vi "Simple Playback Controller.vi"() -> ()   [LabVIEW 2010]
panel:
  out "Joint States":T1(array[cluster])
  in  "Play":bool
  out "Array":T2(array[cluster])
  in  "Done":bool
  in  "Script of positions":i32(listbox)
  in  "Add":bool
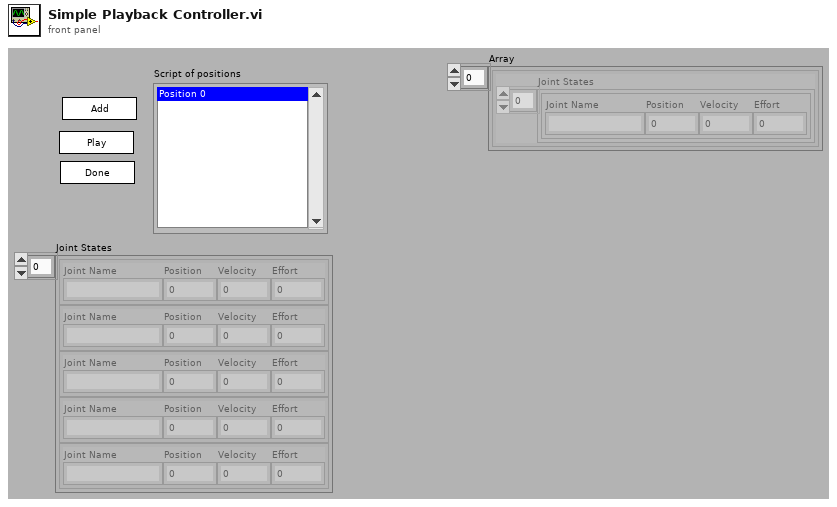
[diagram p1: front panel]
types:
  T1 = cluster{"Joint Name":string, "Position":dbl, "Velocity":dbl, "Effort":dbl}[]
  T2 = cluster{"Joint States":cluster{"Joint Name":string, "Position":dbl, "Velocity":dbl, "Effort":dbl}[]}[]
  T3 = cluster{"Joint States":cluster{"Joint Name":string, "Position":dbl, "Velocity":dbl, "Effort":dbl}[]}
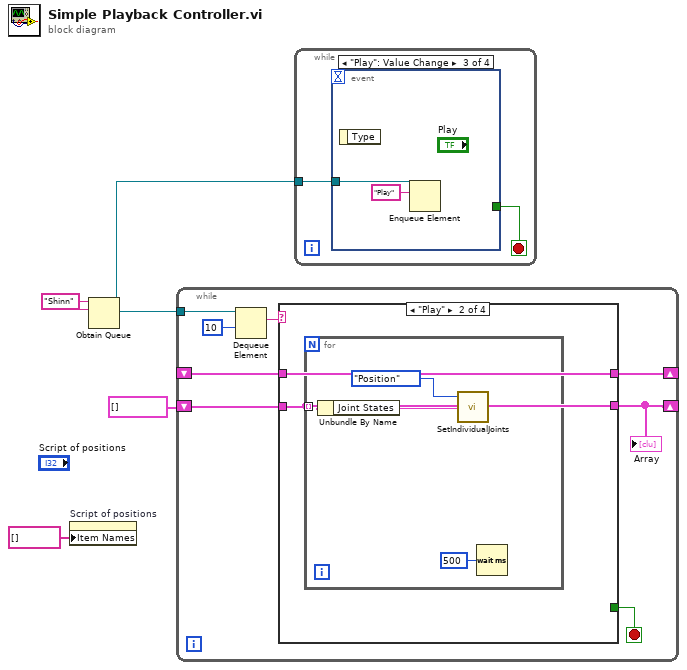
[diagram p0: block diagram]
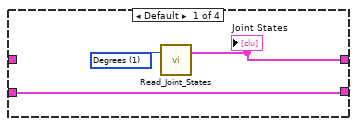
[diagram p2: hidden frame]
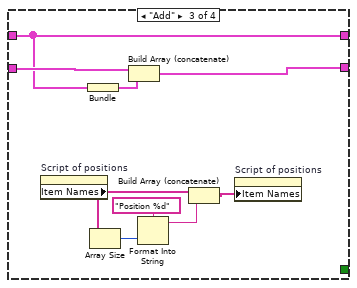
[diagram p3: hidden frame]
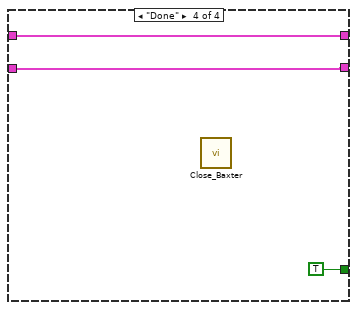
[diagram p4: hidden frame]
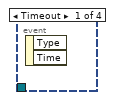
[diagram p5: hidden frame]
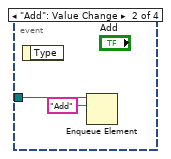
[diagram p6: hidden frame]
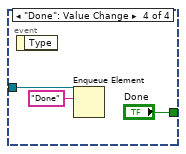
[diagram p7: hidden frame]
diagram:
  w4 = "Shinn" ("name (unnamed)")
  n1 = property on="Script of positions" class="LstBox (strict)"("Item Names"=string[] []) -> ()  [unwired: 2 in, 2 out]
  n2 = Obtain Queue(name (unnamed)=w4, element data type=w4) -> (queue out=w3:refnum<queue>)  [unwired: 3 in, 2 out]
  n3 = while {
    tunnel: w3 -> [w12]
    shift-right: [w8] -> _
    shift-left: _ -> [w7]
    shift-right: [w5] -> _
    shift-left: T2 [] -> [w6]
    stop <- w10 stop-if-true
    n4 = Dequeue Element(queue=w12, timeout in ms (-1)=10) -> (element=w11:string)  [unwired: 1 in, 3 out]
    n5 = case shown="\"Play\"" w11 {
      tunnel: [_ _ _ TRUE] -> w10
      tunnel: [w14 w17 w22 w32] -> w8
      tunnel: w7 -> [_ w17 w22 w32]
      tunnel: [w13 w16 w30 w31] -> w5
      tunnel: w6 -> [w13 w16 w29 w31]
      frame Default {
        w15 = u16 1 items=["Radians", "Degrees"] ("Units (Rad)")
        n6 = call <userlib>:"Read_Joint_States.vi"("Units (deg)"=w15) -> ("Joint States"=w14:T1)  [unwired: 2 in, 1 out]
        "Joint States" <- w14
      }
      frame "Play" {
        n7 = for {
          tunnel: w16 -> [w19] mode=indexing
          n8 = Unbundle By Name(w19) -> ("Joint States"=w18:T1)
          n9 = call <userlib>:"SetIndividualJoints.vi"("Mode"=enum16{"Position", "Velocity", "Effort"}."Position", "Joint States"=w18) -> ()  [unwired: 4 in, 1 out]
          n10 = Wait (ms)(milliseconds to wait=u32 500) -> ()  [unwired: 1 out]
        }
      }
      frame "Add" {
        n11 = property on="Script of positions" class="LstBox (strict)"() -> ("Item Names"=w25:string[])  [unwired: 2 in, 2 out]
        n12 = Bundle("Joint States"=w22) -> (w23:T3)  [unwired: 1 in]
        n13 = Array Size(array=w25) -> (size(s)=w26:i32)
        n14 = Build Array (concatenate)(w29, w23) -> (w30:T2)
        n15 = Format Into String(format string="Position %d" ("name (unnamed)"), w26) -> (resulting string=w27:string)  [unwired: 2 in, 1 out]
        n16 = Build Array (concatenate)(w25, w27) -> (w24:string[])
        n17 = property on="Script of positions" class="LstBox (strict)"("Item Names"=w24) -> ()  [unwired: 2 in, 2 out]
      }
      frame "Done" {
        n18 = call <userlib>:"Close_Baxter.vi"() -> ()  [unwired: 4 in, 1 out]
      }
    }
    "Array" <- w5
  }
  n19 = while {
    tunnel: w3 -> [w34]
    stop <- w35 stop-if-true
    n20 = event shown="[2] \"Play\": Value Change" {
      selector: _ -> [_ _ _ _]
      dyn-events: _ -> [_ _ _ _]
      timeout: _ -> [_ _ _ _]
      tunnel: [_ _ _ "Done"] -> w35
      tunnel: w34 -> [_ w37 w38 w40]
      event Timeout {
        n21 = event-data() -> ()  [unwired: 1 in, 2 out]
      }
      event "Add": Value Change {
        n22 = event-data() -> ()  [unwired: 1 in, 1 out]
        n23 = Enqueue Element(queue=w37, element="Add") -> ()  [unwired: 2 in, 3 out]
      }
      event "Play": Value Change {
        n24 = event-data() -> ()  [unwired: 1 in, 1 out]
        n25 = Enqueue Element(queue=w38, element="Play") -> ()  [unwired: 2 in, 3 out]
      }
      event "Done": Value Change {
        n26 = event-data() -> ()  [unwired: 1 in, 1 out]
        n27 = Enqueue Element(queue=w40, element="Done") -> ()  [unwired: 2 in, 3 out]
      }
    }
  }
